vi "Emballage_BDD_update_PortCom.vi"(8 "Error in":errorcluster caption="Error in (no error)", 10 "champsCom":string, 11 "PortCom":string) -> (0 "Error out":errorcluster)   [LabVIEW 2020]
uses:
  Modules/FS/60_FS_Controles/60_FS_SetGet.ctl
  <vilib>/drjdpowell/SQLite Library/SQL Connection/Open (path).vi
  <vilib>/drjdpowell/SQLite Library/SQL Connection/Open (string).vi
  <vilib>/AdvancedString/Path To Command Line String.vi
  <vilib>/drjdpowell/SQLite Library/SQL Connection/Connection.lvclass
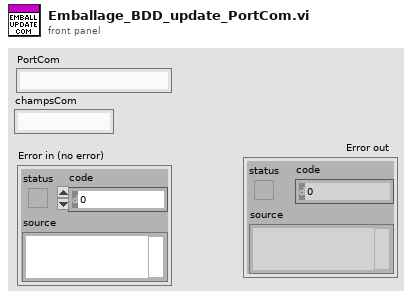
[diagram p1: front panel]
types:
  T1 = typedef "60_FS_SetGet.ctl" = enum16{"set", "get"}
  T2 = typedef "60_FS_CLT_Chemins.ctl" = cluster{"Racine_local":path, "Racine_reseau":path, "Racine_Support_Application":path, "Fichier_Journalisation":path, "Connexion_BDD_VSX":path, "Connexion_BDD_PLZ":path}
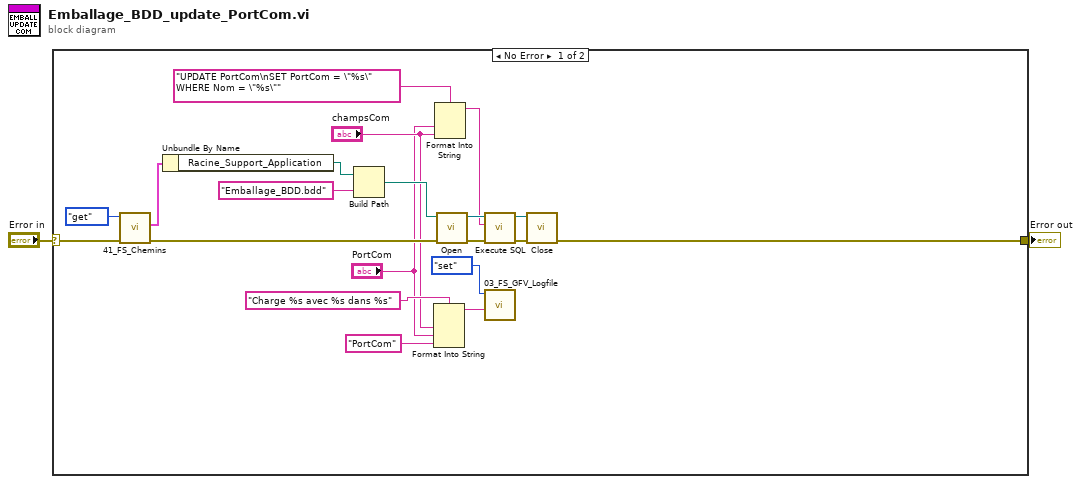
[diagram p0: block diagram]
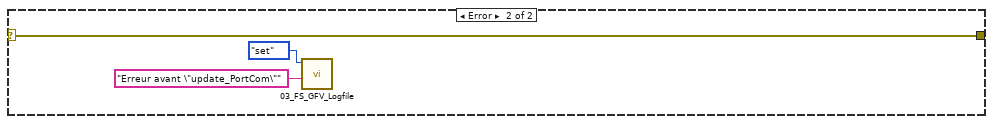
[diagram p2: hidden frame]
diagram:
  n1 = case shown="No Error" "Error in" {
    selector: "Error in" -> [w9 w25]
    tunnel: [w10 w25] -> w2
    frame No Error {
      n2 = call "41_FS_Chemins.vi"("error in (no error)"=w9, "SetGet"=60_FS_SetGet."get") -> ("error out"=w19:errorcluster, "CLT_Chemins_out"=w21:T2)  [unwired: 8 in]
      n3 = Unbundle By Name(w21) -> ("Racine_Support_Application"=w20:path)
      n4 = Build Path(base path=w20, name or relative path="Emballage_BDD.bdd" ("nom ou chemin relatif")) -> (appended path=w12:path)
      n5 = Format Into String(format string="Charge %s avec %s dans %s" ("chaîne de format"), "champsCom", "PortCom", "PortCom" ("entrée 3")) -> (resulting string=w7:string)  [unwired: 2 in, 1 out]
      n6 = Format Into String(format string="UPDATE PortCom\nSET PortCom = \"%s\" WHERE Nom = \"%s\"" ("SQL"), "PortCom", "champsCom") -> (resulting string=w13:string)  [unwired: 2 in, 1 out]
      n7 = call-poly <vilib>:"Open.vi"("error in (no error)"=w19, "db file"=w12) -> ("error out"=w18:errorcluster, "SQLite Connection"=w17:refnum<class "Connection.lvclass">)  [unwired: 8 in]
      n8 = call <vilib>:"Execute SQL.vi"("error in (no error)"=w18, "SQL"=w13, "SQLite Connection in"=w17) -> ("error out"=w16:errorcluster, "SQLite Connection"=w15:refnum<class "Connection.lvclass">)  [unwired: 5 in, 2 out]
      n9 = call "03_FS_GFV_Logfile.vi"("Chaîne"=w7, "States"=60_FS_SetGet."set") -> ()  [unwired: 8 in, 2 out]
      n10 = call-dynamic "Close.vi"("error in (no error)"=w16, "SQLite Connection in"=w15) -> ("error out"=w10:errorcluster)  [unwired: 9 in]
    }
    frame Error {
      n11 = call "03_FS_GFV_Logfile.vi"("Chaîne"="Erreur avant \"update_PortCom\"", "States"=60_FS_SetGet."set") -> ()  [unwired: 8 in, 2 out]
    }
  }
  "Error out" <- w2
